vi "Measure Multiple.vi"(5 "Byte Order (Normal)":T1(ring), 6 "ASCII Precision(6)":i32=6, 7 "Data Format (ASCII)":T2(ring), 8 "error in (no error)":errorcluster, 10 "Measure Count":i32=1, 11 "VISA resource name":refnum<visa-resource-name>) -> (0 "error out":errorcluster, 2 "Data":dbl[](array[numeric]) format="%_6e", 3 "VISA resource name out":refnum<visa-resource-name>)   [LabVIEW 2018, in "Keithley 3706.lvlib"]
uses:
  <instrlib>/Keithley 3706/Keithley 3706.lvlib
panel:
  out "String":string
  out "Output":string
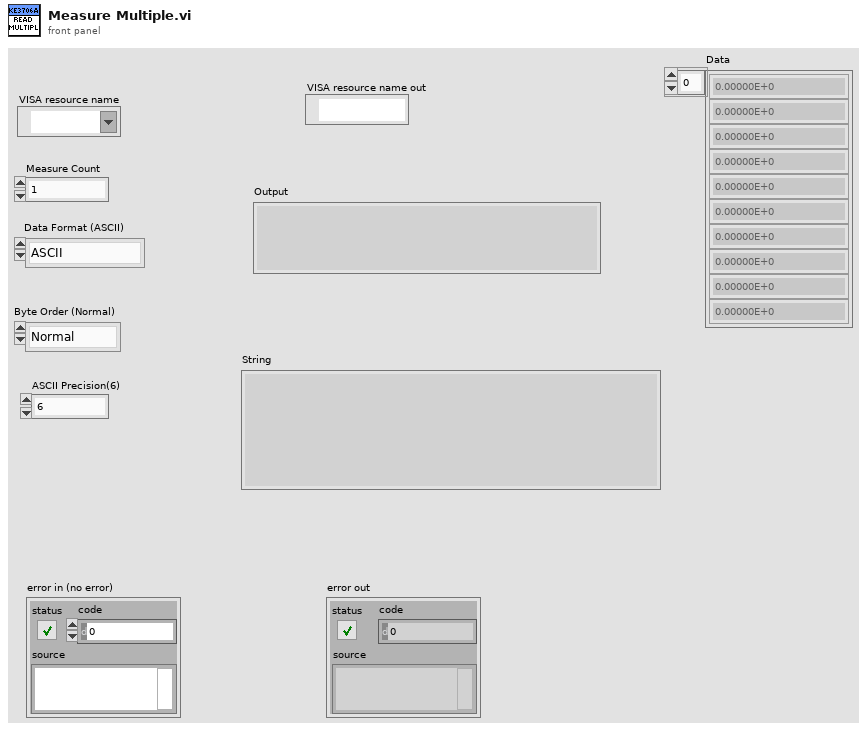
[diagram p1: front panel]
types:
  T1 = enum32{"Normal", "Big Endian", "Little Endian", "Network", "Swapped"}
  T2 = enum32{"ASCII", "Real 32", "Real 64", "Single Precision Real", "Double Precision Real"}
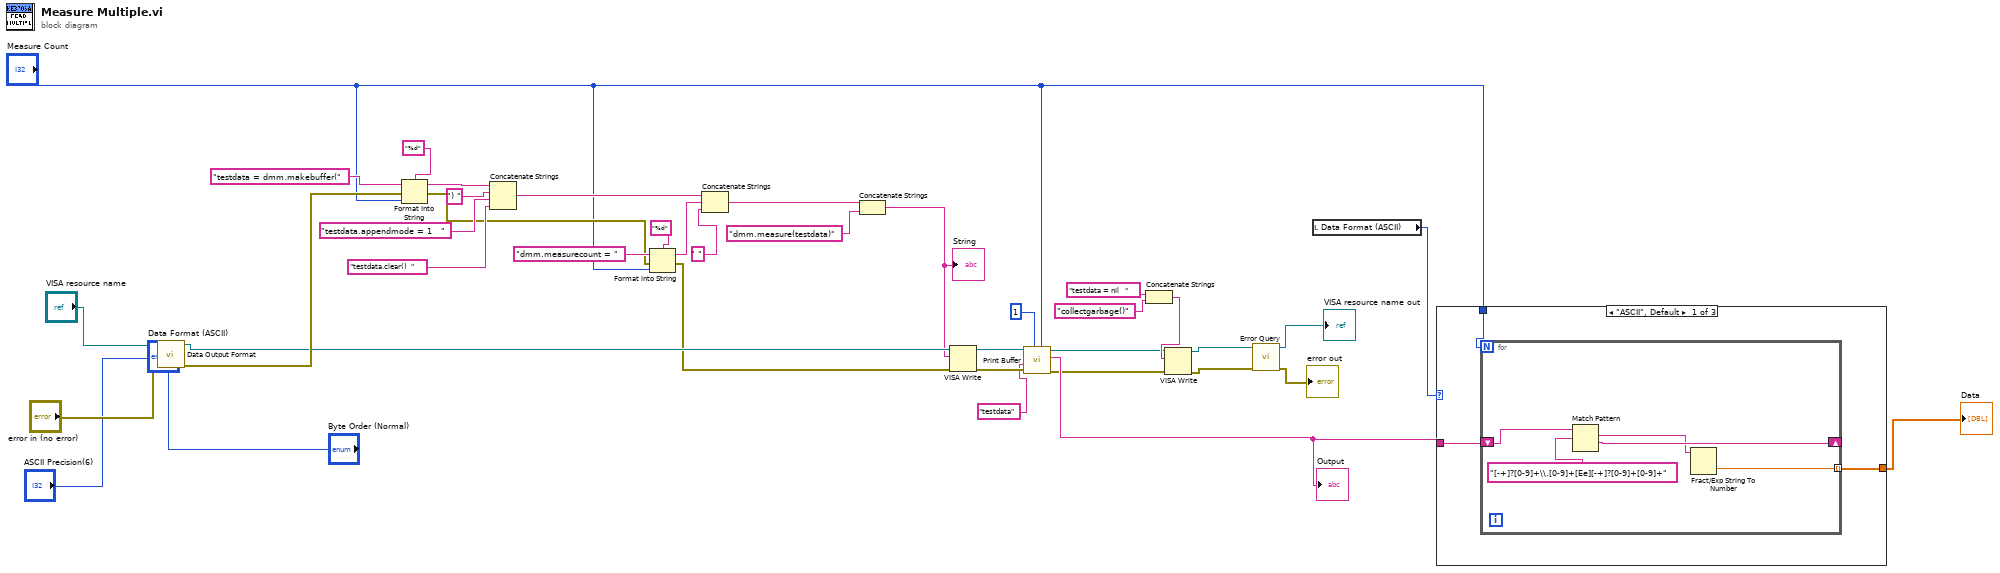
[diagram p0: block diagram]
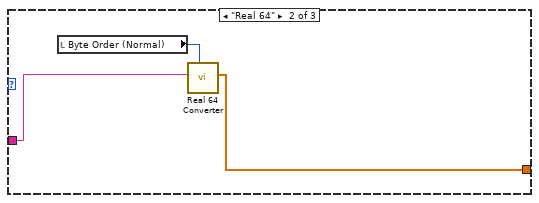
[diagram p2: hidden frame]
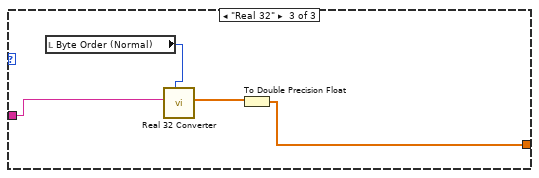
[diagram p3: hidden frame]
diagram:
  n1 = call <instrlib>:"Data Output Format.vi"("Byte Order (Normal)"="Byte Order (Normal)", "error in (no error)"="error in (no error)", "ASCII Precision (6)"="ASCII Precision(6)", "Data Format (ASCII)"="Data Format (ASCII)", "VISA resource name"="VISA resource name") -> ("error out"=w22:errorcluster, "VISA resource name out"=w20:refnum<visa-resource-name>)  [unwired: 5 in]
  n2 = Format Into String(format string="%d", initial string="testdata = dmm.makebuffer(", error in=w22, "Measure Count") -> (resulting string=w33:string, error out=w21:errorcluster)
  n3 = Concatenate Strings(w33, ") ", "testdata.appendmode = 1   ", "testdata.clear()  ") -> (w29:string)
  n4 = Format Into String(format string="%d", initial string="dmm.measurecount = ", error in=w21, "Measure Count") -> (resulting string=w26:string, error out=w19:errorcluster)
  n5 = Concatenate Strings(w29, w26, " ") -> (w24:string)
  n6 = Concatenate Strings(w24, "dmm.measure(testdata)") -> (w9:string)
  "String" <- w9
  n7 = VISA Write(VISA resource name=w20, write buffer=w9, error in (no error)=w19) -> (VISA resource name out=w18:refnum<visa-resource-name>, error out=w17:errorcluster)  [unwired: 1 out]
  n8 = call <instrlib>:"Print Buffer.vi"("End Index (1)"="Measure Count", "Start Index (1)"=1, "error in (no error)"=w17, "Buffer Name(s)"="testdata", "VISA resource name"=w18) -> ("error out"=w3:errorcluster, "Buffer Data"=w8:string, "VISA resource name out"=w4:refnum<visa-resource-name>)  [unwired: 2 in, 2 out]
  "Output" <- w8
  n9 = Concatenate Strings("testdata = nil   ", "collectgarbage()") -> (w5:string)
  n10 = VISA Write(VISA resource name=w4, write buffer=w5, error in (no error)=w3) -> (VISA resource name out=w2:refnum<visa-resource-name>, error out=w1:errorcluster)  [unwired: 1 out]
  n11 = call <instrlib>:"Error Query.vi"("error in (no error)"=w1, "VISA resource name"=w2) -> ("error out"=→"error out":errorcluster, "VISA resource name output"=→"VISA resource name out":refnum<visa-resource-name>)  [unwired: 6 in, 2 out]
  n12 = local read "Data Format (ASCII)"() -> (w12:T2)
  n13 = case shown="\"ASCII\", Default" w12 {
    tunnel: w8 -> [w42 w50 w55]
    tunnel: "Measure Count" -> [w43 _ _]
    tunnel: [w41 w49 w52] -> w10
    frame "ASCII", Default {
      n14 = for {
        N: w43 -> [_]
        shift-right: [w46] -> _
        shift-left: w42 -> [w48]
        tunnel: [w44] -> w41 mode=indexing
        n15 = Match Pattern(string=w48, regular expression="[-+]?[0-9]+\\.[0-9]+[Ee][-+]?[0-9]+[0-9]+") -> (match substring=w45:string, after substring=w46:string)  [unwired: 1 in, 2 out]
        n16 = Fract/Exp String To Number(string=w45) -> (number=w44:dbl)  [unwired: 3 in, 1 out]
      }
    }
    frame "Real 64" {
      n17 = local read "Byte Order (Normal)"() -> (w51:T1)
      n18 = call <instrlib>:"Real 64 Converter.vi"("Byte Order (Normal)"=w51, "Data In"=w50) -> ("Data Array Out"=w49:sgl[])  [unwired: 8 in, 1 out]
    }
    frame "Real 32" {
      n19 = local read "Byte Order (Normal)"() -> (w54:T1)
      n20 = call <instrlib>:"Real 32 Converter.vi"("Byte Order (Normal)"=w54, "Data In"=w55) -> ("Data Array Out"=w53:sgl[])  [unwired: 8 in, 1 out]
      n21 = To Double Precision Float(number=w53) -> (double precision float=w52:dbl[])
    }
  }
  "Data" <- w10
